vi "Plot menu activation GENERAL.vi"(7 "menu tag":string, 8 "error in (no error)":errorcluster, 10 "BluePlotHandle in":refnum<class "RocketPlotHandle.lvclass">, 11 "MenuRef":refnum<k9>) -> (0 "error out":errorcluster, 3 "MenuRef":refnum<k9>)   [LabVIEW 2021, in "RocketPlot.lvlib"]
uses:
  RocketPlot.lvlib
  Classes/RocketPlotHandle/RocketPlotHandle.lvclass
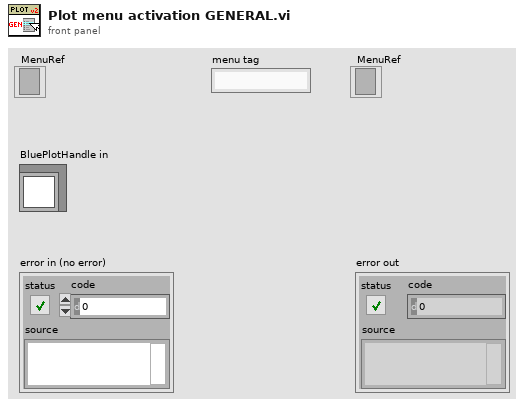
[diagram p1: front panel]
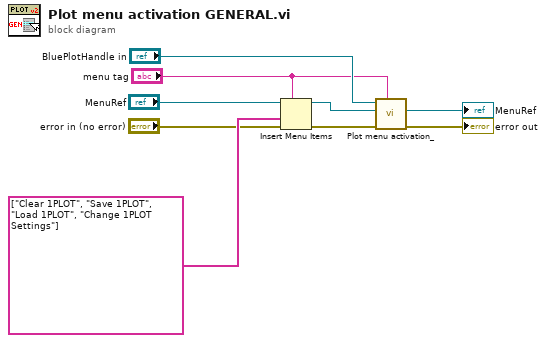
[diagram p0: block diagram]
diagram:
  n1 = Insert Menu Items(5:"menu tag", 6:"error in (no error)", 7:string[] ["Clear 1PLOT", "Save 1PLOT", "Load 1PLOT", "Change 1PLOT Settings"], 9:"MenuRef") -> (0:w6:errorcluster, 3:w5:refnum<k9>)  [unwired: 2 in, 1 out]
  n2 = call-dynamic "Plot menu activation_.vi"("menu tag"="menu tag", "error in (no error)"=w6, "MenuRef"=w5, "BluePlotHandle in"="BluePlotHandle in") -> ("error out"=→"error out":errorcluster, "MenuRef"=→"MenuRef":refnum<k9>)  [unwired: 5 in, 1 out]
